vi "DSF.Shared.Constants.Library Name.Engine.vi"() -> (3 "Engine Library Name":string)   [LabVIEW 2017, in "Data Sharing Framework Engine.lvlib"]
uses:
  Source/Data Sharing Framework Core/Engine/Data Sharing Framework Engine.lvlib
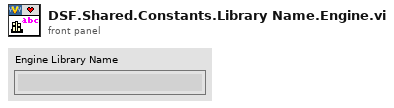
[diagram p1: front panel]
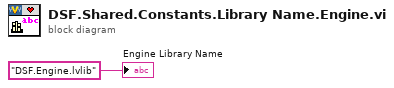
[diagram p0: block diagram]
diagram:
  "Engine Library Name" <- "DSF.Engine.lvlib" ("Library Name")
